vi "RT.Hover.Get__LCR.vi"(4 "error in (no error)":errorcluster, 6 "Container State":T9, 7 "Display State In":T1={"Orientation"=0, "ActivePicture"={"image type"=0, "image depth"=0, "image"=[], "mask"=[], "colors"=[], "Rectangle"={"left"=0, "top"=0, "right"=0, "bottom"=0}}, "Pictures"={"Normal"={"image type"=0, "image depth"=0, "image"=[], "mask"=[], "colors"=[], "Rectangle"={"left"=0, "top"=0, "right"=0, "bottom"=0}}, "Hilite"={"image type"=0, "image depth"=0, "image"=[], "mask"=[], "colors"=[], "Rectangle"={"left"=0, "top"=0, "right"=0, "bottom"=0}}}, "Text"={"String"="", "Font"={"Font Name:"="", "Size"=0, "Strikeout?"=FALSE, "Italic?"=FALSE, "Underline?"=FALSE, "Outline?"=FALSE, "Shadow?"=FALSE, "Bold?"=FALSE}, "TextColor"=0}, "RunTimeSettings"={"Highlight"=FALSE, "ShowButton"=TRUE, "Behaviour"=enum."Switch when pressed", "React if disabled"=FALSE, "Nudge Button"=TRUE, "ShowButton on Hover"=FALSE, "Button Type"=enum."System"}, "Messages"=[], "Status"=0, "XControl Label"="", "Boolean Value"=FALSE} {"Status" format="%.0x"}) -> (0 "error out":errorcluster, 2 "Value":bool, 3 "Display State Out":T1={"Orientation"=0, "ActivePicture"={"image type"=0, "image depth"=0, "image"=[], "mask"=[], "colors"=[], "Rectangle"={"left"=0, "top"=0, "right"=0, "bottom"=0}}, "Pictures"={"Normal"={"image type"=0, "image depth"=0, "image"=[], "mask"=[], "colors"=[], "Rectangle"={"left"=0, "top"=0, "right"=0, "bottom"=0}}, "Hilite"={"image type"=0, "image depth"=0, "image"=[], "mask"=[], "colors"=[], "Rectangle"={"left"=0, "top"=0, "right"=0, "bottom"=0}}}, "Text"={"String"="", "Font"={"Font Name:"="", "Size"=0, "Strikeout?"=FALSE, "Italic?"=FALSE, "Underline?"=FALSE, "Outline?"=FALSE, "Shadow?"=FALSE, "Bold?"=FALSE}, "TextColor"=0}, "RunTimeSettings"={"Highlight"=FALSE, "ShowButton"=TRUE, "Behaviour"=enum."Switch when pressed", "React if disabled"=FALSE, "Nudge Button"=TRUE, "ShowButton on Hover"=FALSE, "Button Type"=enum."System"}, "Messages"=[], "Status"=0, "XControl Label"="", "Boolean Value"=FALSE} {"Status" format="%.0x"})   [LabVIEW 2011, in "BooleanXControl__LCR.xctl"]
uses:
  BooleanXControl__LCR.xctl
  <vilib>/_xctls/Container State.ctl
  Abilities/BX.State__LCR.ctl
  Controls/BX.Orientation__LCR.ctl
  <vilib>/picture/picture.llb/imagedata.ctl
  Controls/BX.RTSettings__LCR.ctl
  Controls/BX.Behaviour__LCR.ctl
  Controls/BX.ButtonType__LCR.ctl
  Controls/BX.Message__LCR.ctl
  Controls/BX.Commands__LCR.ctl
  <vilib>/_xctls/XControlSupport.lvlib
panel:
  # "Replace the Value Indicator below with an Indicator of desired type.\nDo not remove this Indicator or the others from the connector pane. \nDo not change the connector pane pattern.\nThe Value Indicator should always be the second terminal from top on the output side in the connector pane."
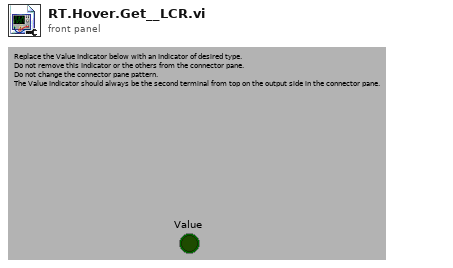
[diagram p1: front panel]
types:
  T1 = typedef "BooleanXControl__LCR.xctl/BX.State__LCR.ctl" = cluster{"Orientation":T2, "ActivePicture":T3, "Pictures":cluster{"Normal":T3, "Hilite":T3}, "Text":cluster{"String":string, "Font":cluster{"Font Name:":string, "Size":i16, "Strikeout?":bool, "Italic?":bool, "Underline?":bool, "Outline?":bool, "Shadow?":bool, "Bold?":bool}, "TextColor":u32}, "RunTimeSettings":T4, "Messages":T7[], "Status":u16, "XControl Label":string, "Boolean Value":bool}
  T2 = typedef "BooleanXControl__LCR.xctl/BX.Orientation__LCR.ctl" = u8
  T3 = typedef "imagedata.ctl" = cluster{"image type":i32, "image depth":i32, "image":u8[], "mask":u8[], "colors":u32[], "Rectangle":cluster{"left":i16, "top":i16, "right":i16, "bottom":i16}}
  T4 = typedef "BooleanXControl__LCR.xctl/BX.RTSettings__LCR.ctl" = cluster{"Highlight":bool, "ShowButton":bool, "Behaviour":T5, "React if disabled":bool, "Nudge Button":bool, "ShowButton on Hover":bool, "Button Type":T6}
  T5 = typedef "BooleanXControl__LCR.xctl/BX.Behaviour__LCR.ctl" = enum16{"Switch when pressed", "Switch when released", "Switch until released"}
  T6 = typedef "BooleanXControl__LCR.xctl/BX.ButtonType__LCR.ctl" = enum16{"System", "Modern", "Classic", "Decoration"}
  T7 = typedef "BooleanXControl__LCR.xctl/BX.Message__LCR.ctl" = cluster{"Command":T8, "Parameter":variant}
  T8 = typedef "BooleanXControl__LCR.xctl/BX.Commands__LCR.ctl" = enum16{"None", "SetPicture", "SetFont", "SetText", "SetOrientation", "Redraw", "SetTextColor", "SetRTSettings", "MultipleUpdate", "RT.Button", "RT.Hilite", "RT.Behaviour", "RT.Disabled", "ShowGUI", "RT.Nudge", "RT.Hover", "RT.ButtonType"}
  T9 = typedef "XControlSupport.lvlib/Container State.ctl" = cluster{"Indicator?":bool, "Run Mode?":bool, " Refnum":refnum<vi>}
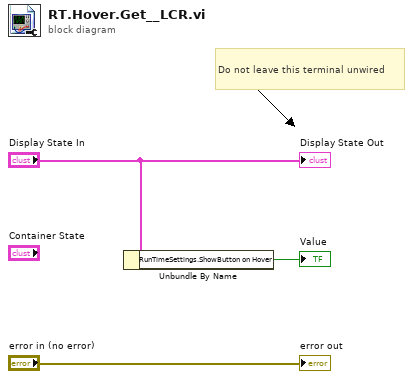
[diagram p0: block diagram]
diagram:
  # "Do not leave this terminal unwired"
  n1 = Unbundle By Name("Display State In") -> ("RunTimeSettings.ShowButton on Hover"=→"Value":bool)
  "error out" <- "error in (no error)"
  "Display State Out" <- "Display State In"
